vi "Get Legend String.vi"(7 "Initial String":string="Slice ", 9 "Pair Array Length":i32, 11 "Color Pair Array In":cluster{"Color":u32, "String":string}[](array[cluster])) -> (3 "Color Pair Array Out":cluster{"Color":u32, "String":string}[](array[cluster]))   [LabVIEW 2020, in "3D Plot.lvclass"]
uses:
  3D Plot.lvclass
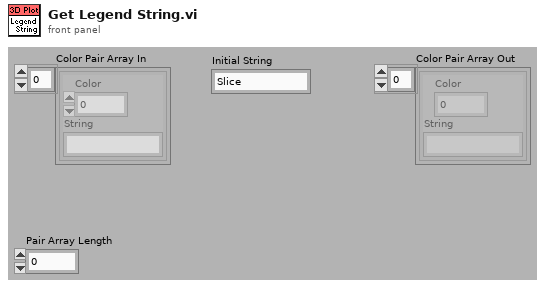
[diagram p1: front panel]
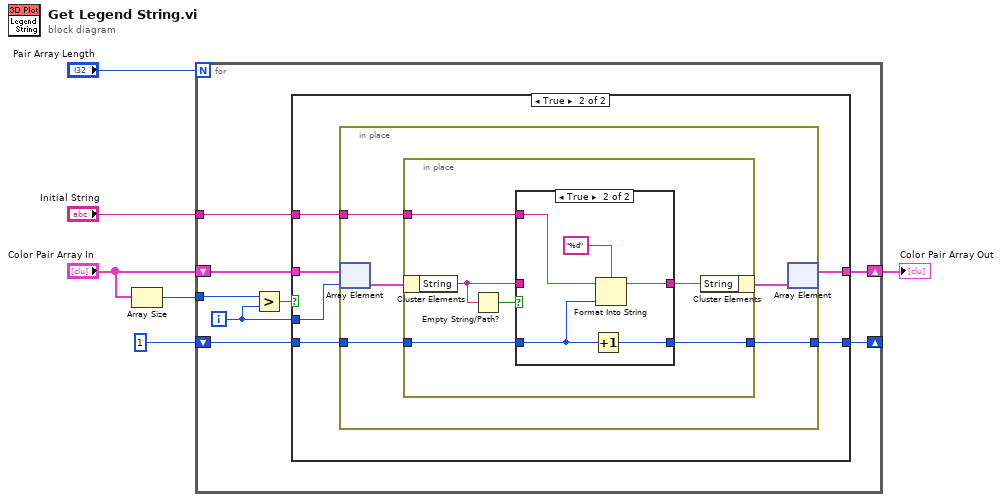
[diagram p0: block diagram]
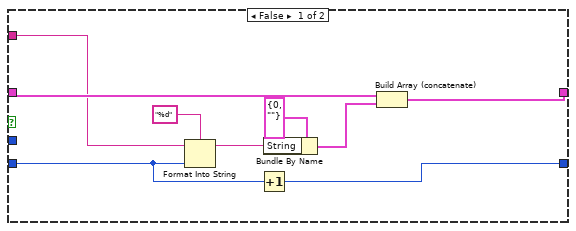
[diagram p2: hidden frame]
diagram:
  n1 = Array Size(array="Color Pair Array In") -> (size(s)=w2:i32)
  n2 = for {
    N: "Pair Array Length" -> [_]
    shift-right: [w13] -> _
    shift-left: u8 1 -> [w14]
    tunnel: "Initial String" -> [w12]
    tunnel: w2 -> [w9]
    shift-right: [w7] -> w1
    shift-left: "Color Pair Array In" -> [w11]
    i -> [w8]
    n3 = Greater?(x=w9, y=w8) -> (0:w10:bool)
    n4 = case shown="True" w10 {
      tunnel: w14 -> [w17 w29]
      tunnel: [w16 w28] -> w13
      tunnel: w12 -> [w19 w27]
      tunnel: w11 -> [w23 w26]
      tunnel: w8 -> [_ w25]
      tunnel: [w22 w24] -> w7
      frame False {
        n5 = Format Into String(format string="%d", initial string=w19, w17) -> (resulting string=w18:string)  [unwired: 1 in, 1 out]
        n6 = Increment(x=w17) -> (x+1=w16:u8)
        n7 = Bundle By Name(cluster=cluster{"Color":u32, "String":string} {"Color"=0, "String"=""} ("Color Pair"), "String"=w18) -> (w15:cluster{"Color":u32, "String":string})
        n8 = Build Array (concatenate)(w23, w15) -> (w22:cluster{"Color":u32, "String":string}[])
      }
      frame True {
        n9 = in-place {
          in-place-border: w29 -> [w34]
          in-place-border: [w33] -> w28
          in-place-border: w27 -> [w32]
          n10 = in-place-array #1(w26, w25) -> (w31:cluster{"Color":u32, "String":string})
          n11 = in-place {
            in-place-border: w34 -> [w40]
            in-place-border: [w39] -> w33
            in-place-border: w32 -> [w35]
            n12 = in-place-cluster #2(w31) -> ("String"=w37:string)
            n13 = Empty String/Path?(string/path=w37) -> (empty?=w38:bool)
            n14 = case shown="True" w38 {
              tunnel: w40 -> [w41 w46]
              tunnel: [w41 w45] -> w39
              tunnel: [w42 w44] -> w36
              tunnel: w37 -> [w42 _]
              tunnel: w35 -> [_ w43]
              frame False {
              }
              frame True {
                n15 = Increment(x=w46) -> (x+1=w45:u8)
                n16 = Format Into String(format string="%d", initial string=w43, w46) -> (resulting string=w44:string)  [unwired: 1 in, 1 out]
              }
            }
            n17 = in-place-cluster #2("String"=w36) -> (w30:cluster{"Color":u32, "String":string})
          }
          n18 = in-place-array #1(w30) -> (w24:cluster{"Color":u32, "String":string}[])  [unwired: 1 out]
        }
      }
    }
  }
  "Color Pair Array Out" <- w1
